vi "Main.vi"() -> ()   [LabVIEW 2014]
doc: "The boiler controller allows a user to start and shut down a boiler.\n\nUse the Reset, Start, and Light Pilot controls to sequentially start the boiler. \nUse the Fuel Control Valve to change the flow of fuel into the boiler. \nUse the Stop Boiler button to shut down the boiler. \nTo shut down the system or in the event of an emergency, use the Emergency Stop button to close the application completely."
uses:
  controls/MHL Data.ctl
  controls/MHL UI Data.ctl
  controls/MHL Status.ctl
  controls/MHL References.ctl
  controls/MHL Configuration.ctl
  support/Boiler System Globals.vi
  <vilib>/Utility/error.llb/Error Cluster From Error Code.vi
  <vilib>/ErrorRing/Error Ring.xnode
  support/Message Queue/Message Queue.lvlib
  support/User Event - Stop/User Event - Stop.lvlib
  Controller/Controller.lvlib
  Boiler/Boiler.lvlib
panel:
  in  "Fuel Control Valve":u32(slide) min=10 max=75 scale=10.0..75.0
  in  "Stop Boiler":bool
  in  "Light Pilot":bool
  out "Forced Draft Fan":bool
  out "Pilot":bool
  out "Pilot Gas Valve":bool
  out "Primary Fan":bool
  out "Status":string
  in  "Start":bool
  in  "Reset":bool
  in  "Emergency Stop":bool
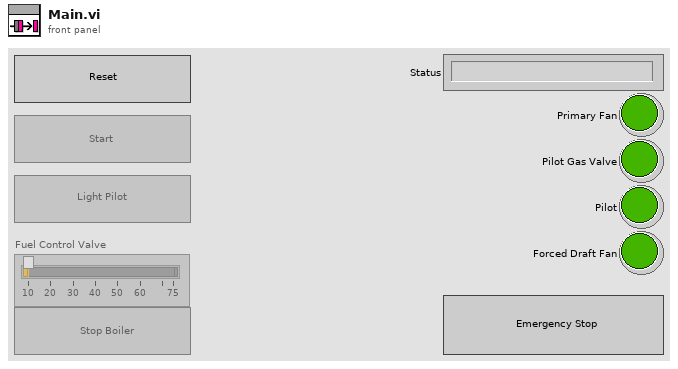
[diagram p1: front panel]
types:
  T1 = typedef "MHL Data.ctl" = cluster{"MHL User Interface Data":T2, "MHL References":T4, "MHL Configuration":T5}
  T2 = typedef "MHL UI Data.ctl" = cluster{"Status":string, "Fuel Control Valve":u32, "Primary Fan":bool, "Pilot Gas Valve":bool, "Pilot":bool, "Forced Draft Fan":bool, "MHL Status":T3}
  T3 = typedef "MHL Status.ctl" = enum16{"Lockout", "Ready", "Pre-Purge", "Pre-Purge Complete", "Pilot On", "Boiler Running", "Shutdown", "Purge"}
  T4 = typedef "MHL References.ctl" = cluster{"Reset Ref":refnum<vi>, "Start Ref":refnum<vi>, "Light Pilot Ref":refnum<vi>, "Stop Boiler Ref":refnum<vi>, "Fuel Control Valve Ref":refnum<vi>}
  T5 = typedef "MHL Configuration.ctl" = cluster{"Fuel Control Valve Maximum":dbl, "Fuel Control Valve Minimum":dbl}
  T6 = typedef "Configuration Data.ctl" = cluster{"MHL Configuration":T5, "Controller Configuration":T7, "Boiler Configuration":T8}
  T7 = typedef "Controller.lvlib/Controller Configuration.ctl" = cluster{"Purge Time":u32, "Flame Threshold":u32}
  T8 = typedef "Boiler.lvlib/Boiler Configuration.ctl" = cluster{"Pilot Increment (ms)":u32, "Pilot Decrement (ms)":u32}
  T9 = typedef "Notifiers.ctl" = cluster{"Handshake":refnum<notifier>, "Flame Level":refnum<notifier>, "Controller Exit":refnum<notifier>, "Boiler Exit":refnum<notifier>}
  T10 = typedef "Message Queue.lvlib/All Message Queues.ctl" = cluster{"MHL":refnum<queue>, "Boiler Controller":refnum<queue>, "Boiler":refnum<queue>}
  T11 = enum16{"open", "replace", "create", "open or create", "replace or create", "replace or create with confirmation"}
  T12 = enum32{"invalid app kind", "Development System", "Run Time System", "Student Edition", "Embedded LabVIEW", "Evaluation", "Custom"}
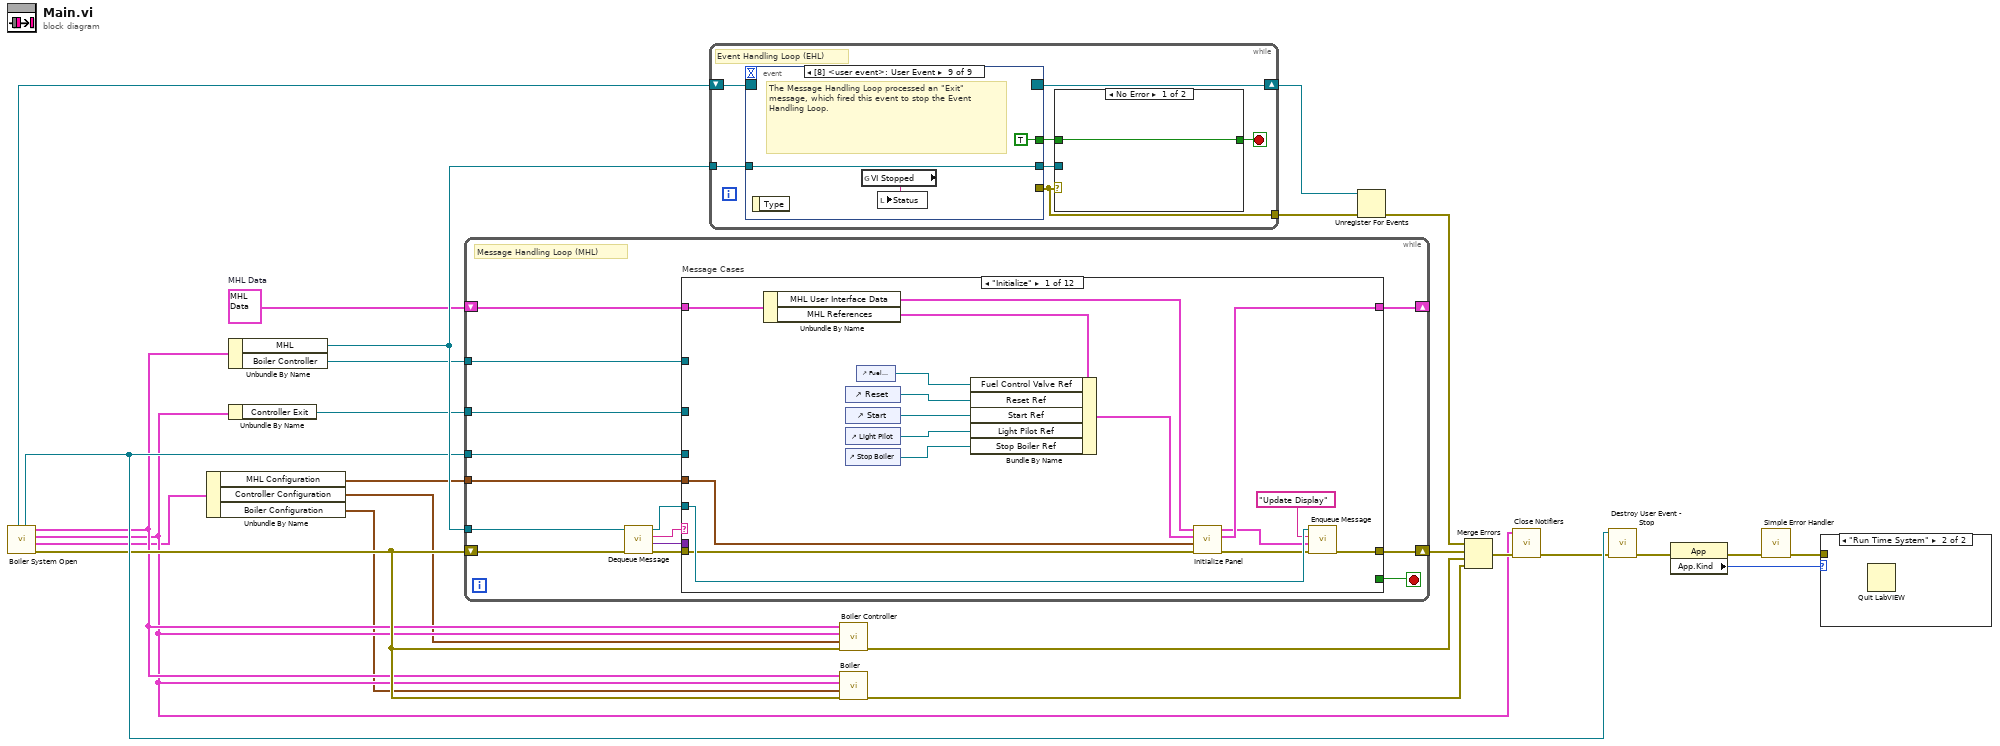
[diagram p0: block diagram]
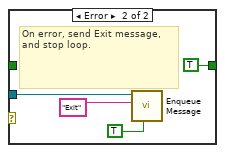
[diagram p3: hidden frame]
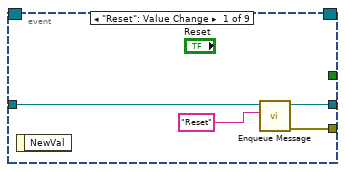
[diagram p4: hidden frame]
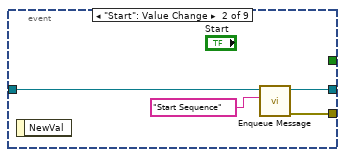
[diagram p5: hidden frame]
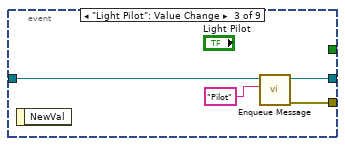
[diagram p6: hidden frame]
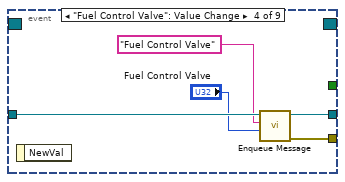
[diagram p7: hidden frame]
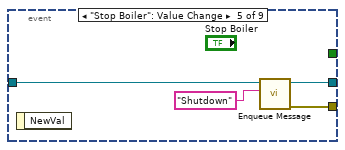
[diagram p8: hidden frame]
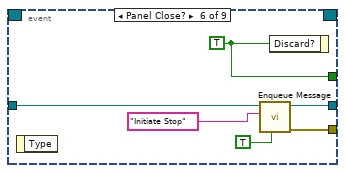
[diagram p9: hidden frame]
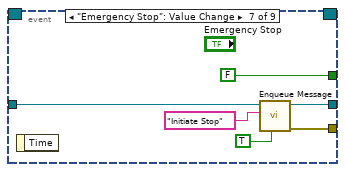
[diagram p10: hidden frame]
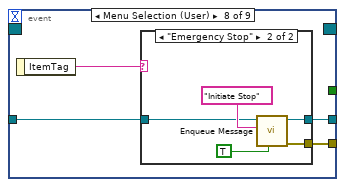
[diagram p11: hidden frame]
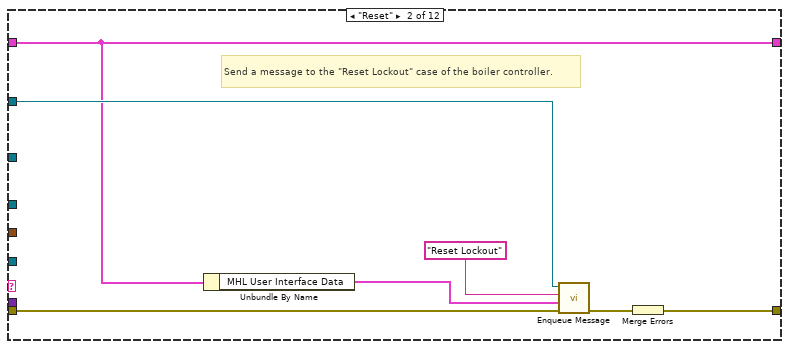
[diagram p13: hidden frame]
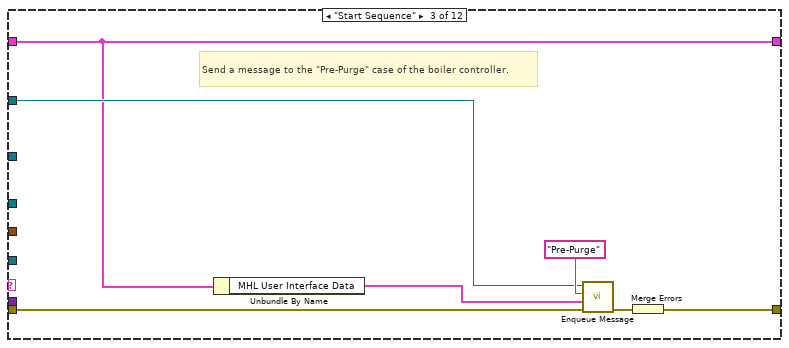
[diagram p14: hidden frame]
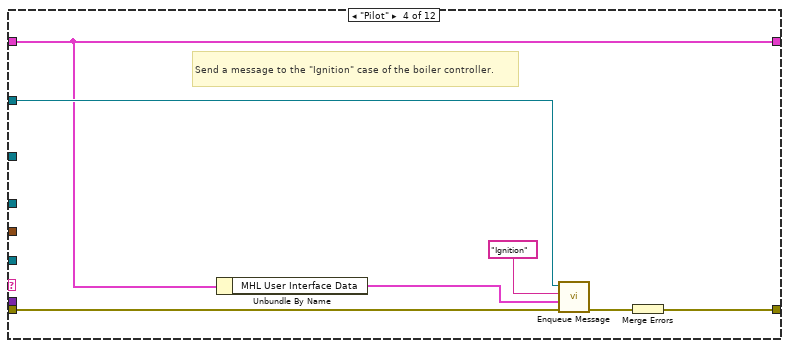
[diagram p15: hidden frame]
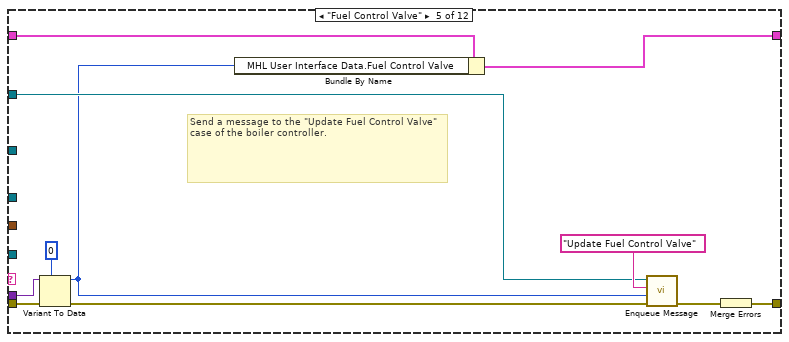
[diagram p16: hidden frame]
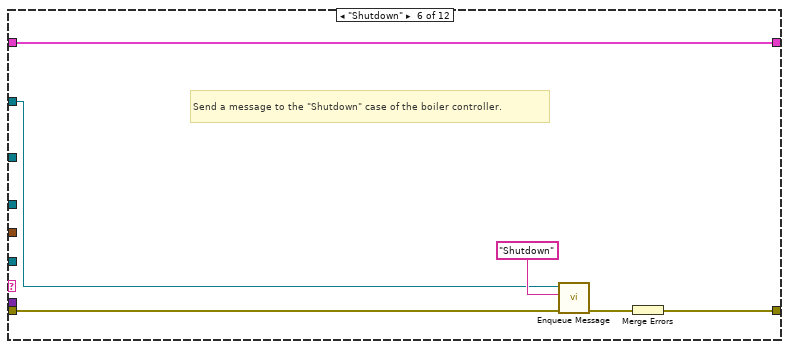
[diagram p17: hidden frame]
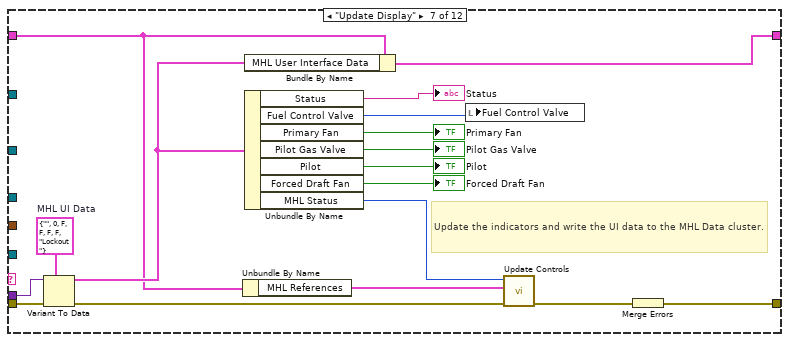
[diagram p18: hidden frame]
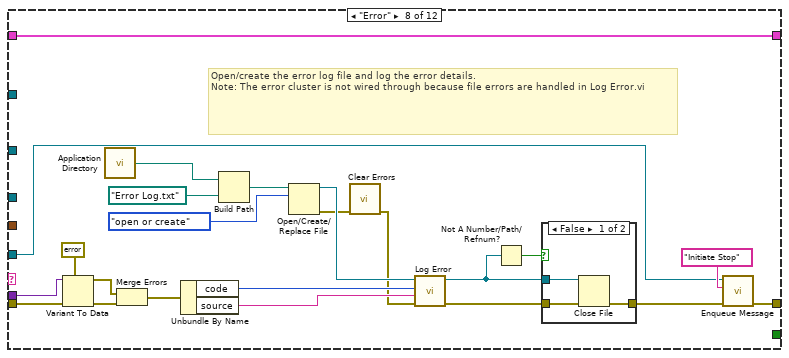
[diagram p19: hidden frame]
diagram:
  w19 = T1 {"MHL User Interface Data"={"Status"="", "Fuel Control Valve"=0, "Primary Fan"=FALSE, "Pilot Gas Valve"=FALSE, "Pilot"=FALSE, "Forced Draft Fan"=FALSE, "MHL Status"=enum."Lockout"}, "MHL References"={"Reset Ref"=refnum, "Start Ref"=refnum, "Light Pilot Ref"=refnum, "Stop Boiler Ref"=refnum, "Fuel Control Valve Ref"=refnum}, "MHL Configuration"={"Fuel Control Valve Maximum"=0.0, "Fuel Control Valve Minimum"=0.0}}  # MHL Data
  n1 = call "Boiler System Open.vi"() -> ("error out"=w10:errorcluster, "Configuration Data"=w4:T6, "Notifiers"=w5:T9, "Message Queues"=w9:T10, "User Event - Stop"=w12:refnum<user-event>, "Stop Event Registration Refnum"=w13:refnum<event-registration>)  [unwired: 6 in]
  n2 = Unbundle By Name(w4) -> ("MHL Configuration"=w3:T5, "Controller Configuration"=w2:T7, "Boiler Configuration"=w1:T8)
  n3 = Unbundle By Name(w9) -> ("MHL"=w24:refnum<queue>, "Boiler Controller"=w17:refnum<queue>)
  n4 = Unbundle By Name(w5) -> ("Controller Exit"=w11:refnum<notifier>)
  n5 = while {
    tunnel: w24 -> [w29]
    shift-right: [w38] -> _
    shift-left: w19 -> [w39]
    tunnel: w12 -> [w35]
    shift-right: [w36] -> w25
    shift-left: w10 -> [w34]
    tunnel: w17 -> [w28]
    tunnel: w11 -> [w27]
    tunnel: w3 -> [w26]
    stop <- w37 stop-if-true
    # "Message Handling Loop (MHL)"
    n6 = call "Dequeue Message.vi"("error in (no error)"=w34, "Message Queue"=w29) -> ("error out"=w33:errorcluster, "Message Data"=w31:variant, "Message"=w32:string, "dup Message Queue"=w30:refnum<queue>)  [unwired: 6 in]
    n7 = case "Message Cases" shown="\"Initialize\"" w32 {
      selector: w32 -> [_ _ _ _ _ _ _ _ _ _ _ w172]
      tunnel: w30 -> [w49 _ _ _ _ _ _ w120 w141 w148 w170 _]
      tunnel: w33 -> [w43 w62 w69 w76 w84 w92 w110 w118 w146 w150 w163 _]
      tunnel: [w50 w63 w70 w77 w88 w93 w111 w116 w143 w149 w166 w171] -> w36
      tunnel: w39 -> [w51 w58 w65 w72 w79 w94 w96 w134 w145 w154 w169 w173]
      tunnel: [w41 w58 w65 w72 w78 w94 w100 w134 w145 w154 w169 w173] -> w38
      tunnel: [_ _ _ _ _ _ _ _ _ _ TRUE _] -> w37
      tunnel: w31 -> [_ _ _ _ w82 _ w109 w117 _ _ _ _]
      tunnel: w35 -> [_ _ _ _ _ _ _ _ _ _ w165 _]
      tunnel: w28 -> [_ w59 w66 w73 w85 w89 _ _ w142 _ _ _]
      tunnel: w27 -> [_ _ _ _ _ _ _ _ _ w147 _ _]
      tunnel: w26 -> [w47 _ _ _ _ _ _ _ _ _ _ _]
      frame "Initialize" {
        n8 = Unbundle By Name(w51) -> ("MHL User Interface Data"=w44:T2, "MHL References"=w45:T4)
        n9 = control-ref of="Reset"() -> (w53:refnum<vi>)
        n10 = control-ref of="Start"() -> (w54:refnum<vi>)
        n11 = control-ref of="Light Pilot"() -> (w55:refnum<vi>)
        n12 = control-ref of="Stop Boiler"() -> (w56:refnum<vi>)
        n13 = control-ref of="Fuel Control Valve"() -> (w52:refnum<vi>)
        n14 = Bundle By Name(cluster=w45, "Fuel Control Valve Ref"=w52, "Reset Ref"=w53, "Start Ref"=w54, "Light Pilot Ref"=w55, "Stop Boiler Ref"=w56) -> (w46:T4)
        n15 = call "Initialize Panel.vi"("error in"=w43, "MHL Configuration"=w47, "MHL References"=w46, "MHL UI Data in"=w44) -> ("error out"=w42:errorcluster, "MHL Data out"=w41:T1, "MHL UI Data out"=w40:T2)  [unwired: 5 in]
        n16 = call "Enqueue Message.vi"("error in (no error)"=w42, "Message Data"=w40, "Message"="Update Display", "Message Queue"=w49) -> ("error out"=w50:errorcluster)  [unwired: 6 in, 1 out]
      }
      frame "Reset" {
        # "Send a message to the \"Reset Lockout\" case of the boiler controller."
        n17 = Unbundle By Name(w58) -> ("MHL User Interface Data"=w57:T2)
        n18 = call "Enqueue Message.vi"("error in (no error)"=w62, "Message Data"=w57, "Message"="Reset Lockout", "Message Queue"=w59) -> ("error out"=w61:errorcluster)  [unwired: 6 in, 1 out]
        n19 = Merge Errors(w61) -> (w63:errorcluster)
      }
      frame "Start Sequence" {
        # "Send a message to the \"Pre-Purge\" case of the boiler controller."
        n20 = Unbundle By Name(w65) -> ("MHL User Interface Data"=w64:T2)
        n21 = call "Enqueue Message.vi"("error in (no error)"=w69, "Message Data"=w64, "Message"="Pre-Purge", "Message Queue"=w66) -> ("error out"=w68:errorcluster)  [unwired: 6 in, 1 out]
        n22 = Merge Errors(w68) -> (w70:errorcluster)
      }
      frame "Pilot" {
        # "Send a message to the \"Ignition\" case of the boiler controller."
        n23 = Unbundle By Name(w72) -> ("MHL User Interface Data"=w71:T2)
        n24 = call "Enqueue Message.vi"("error in (no error)"=w76, "Message Data"=w71, "Message"="Ignition", "Message Queue"=w73) -> ("error out"=w75:errorcluster)  [unwired: 6 in, 1 out]
        n25 = Merge Errors(w75) -> (w77:errorcluster)
      }
      frame "Fuel Control Valve" {
        # "Send a message to the \"Update Fuel Control Valve\" case of the boiler controller."
        n26 = Variant To Data(error in=w84, type=u32 0 ("Fuel Control Valve"), Variant=w82) -> (data=w80:u32, error out=w83:errorcluster)
        n27 = Bundle By Name(cluster=w79, "MHL User Interface Data.Fuel Control Valve"=w80) -> (w78:T1)
        n28 = call "Enqueue Message.vi"("error in (no error)"=w83, "Message Data"=w80, "Message"="Update Fuel Control Valve", "Message Queue"=w85) -> ("error out"=w87:errorcluster)  [unwired: 6 in, 1 out]
        n29 = Merge Errors(w87) -> (w88:errorcluster)
      }
      frame "Shutdown" {
        # "Send a message to the \"Shutdown\" case of the boiler controller."
        n30 = call "Enqueue Message.vi"("error in (no error)"=w92, "Message"="Shutdown", "Message Queue"=w89) -> ("error out"=w91:errorcluster)  [unwired: 7 in, 1 out]
        n31 = Merge Errors(w91) -> (w93:errorcluster)
      }
      frame "Update Display" {
        w108 = T2 {"Status"="", "Fuel Control Valve"=0, "Primary Fan"=FALSE, "Pilot Gas Valve"=FALSE, "Pilot"=FALSE, "Forced Draft Fan"=FALSE, "MHL Status"=enum."Lockout"}  # MHL UI Data
        # "Update the indicators and write the UI data to the MHL Data cluster."
        n32 = Variant To Data(error in=w110, type=w108, Variant=w109) -> (data=w101:T2, error out=w99:errorcluster)
        n33 = Unbundle By Name(w96) -> ("MHL References"=w95:T4)
        n34 = Bundle By Name(cluster=w96, "MHL User Interface Data"=w101) -> (w100:T1)
        n35 = Unbundle By Name(w101) -> ("Status"=→"Status":string, "Fuel Control Valve"=w106:u32, "Primary Fan"=→"Primary Fan":bool, "Pilot Gas Valve"=→"Pilot Gas Valve":bool, "Pilot"=→"Pilot":bool, "Forced Draft Fan"=→"Forced Draft Fan":bool, "MHL Status"=w97:T3)
        n36 = local write "Fuel Control Valve"(w106) -> ()
        n37 = call "Update Controls.vi"("error in"=w99, "MHL References"=w95, "MHL Status"=w97) -> ("error out"=w98:errorcluster)  [unwired: 8 in]
        n38 = Merge Errors(w98) -> (w111:errorcluster)
      }
      frame "Error" {
        # "Open/create the error log file and log the error details.\nNote: The error cluster is not wired through because file errors are handled in Log Error.vi"
        n39 = Variant To Data(error in=w118, type=errorcluster {"status"=FALSE, "code"=0, "source"=""} ("error out"), Variant=w117) -> (data=w130:errorcluster, error out=w131:errorcluster)
        n40 = call <vilib>:"Application Directory.vi"() -> ("Application Directory"=w128:path)
        n41 = Merge Errors(w130, w131) -> (w129:errorcluster)
        n42 = Unbundle By Name(w129) -> ("code"=w123:i32, "source"=w122:string)
        n43 = Build Path(base path=w128, name or relative path=path "Error Log.txt") -> (appended path=w127:path)
        n44 = Open/Create/Replace File(file path (use dialog)=w127, operation (0:open)=T11."open or create") -> (refnum out=w125:refnum<file>, error out=w113:errorcluster)  [unwired: 4 in, 1 out]
        n45 = call <vilib>:"Clear Errors.vi"("error in (no error)"=w113) -> ("error out"=w112:errorcluster)  [unwired: 5 in, 1 out]
        n46 = call "Log Error.vi"("error in"=w112, "Source"=w122, "Code"=w123, "Error Log Refnum In"=w125) -> ("error out"=w124:errorcluster, "Error Log Refnum Out"=w115:refnum<file>)  [unwired: 6 in]
        n47 = Not A Number/Path/Refnum?(number/path/refnum=w115) -> (NaN/Path/Refnum?=w114:bool)
        n48 = case shown="False" w114 {
          tunnel: w124 -> [w137 w138]
          tunnel: w115 -> [w136 _]
          tunnel: [w135 w138] -> w121
          frame False {
            n49 = Close File(refnum=w136, error in=w137) -> (error out=w135:errorcluster)  [unwired: 1 out]
          }
          frame True {
          }
        }
        n50 = call "Enqueue Message.vi"("error in (no error)"=w121, "Message"="Initiate Stop", "Message Queue"=w120) -> ("error out"=w116:errorcluster)  [unwired: 7 in, 1 out]
      }
      frame "Initiate Stop" {
        # "When stopping, first send a message to stop the boiler controller. Then wait for the boiler and boiler controller to exit."
        n51 = call "Enqueue Message.vi"("error in (no error)"=w146, "Message"="Exit", "Message Queue"=w142) -> ("error out"=w144:errorcluster)  [unwired: 7 in, 1 out]
        n52 = call "Enqueue Message.vi"("error in (no error)"=w144, "Message"="Wait on Boiler Exit", "Message Queue"=w141) -> ("error out"=w143:errorcluster)  [unwired: 7 in, 1 out]
      }
      frame "Wait on Boiler Exit" {
        # "Monitor the boiler controller to determine if it has completed its Exit. Wait 10 milliseconds for the boiler controller to respond. \nIf the notification does not occur, then enqueue another Wait on Boiler Exit message.\nIf the notification occurs, then exit the Message Handling Loop."
        n53 = Wait on Notification(notifier=w147, timeout in ms (-1)=10, error in (no error)=w150) -> (timed out?=w152:bool, error out=w151:errorcluster)  [unwired: 1 in, 2 out]
        n54 = case shown="True" w152 {
          tunnel: w151 -> [w158 w162]
          tunnel: w148 -> [w157 w160]
          tunnel: [w155 w161] -> w149
          frame False {
            n55 = call "Enqueue Message.vi"("error in (no error)"=w158, "Message"="Exit", "Message Queue"=w157) -> ("error out"=w155:errorcluster)  [unwired: 7 in, 1 out]
          }
          frame True {
            n56 = call "Enqueue Message.vi"("error in (no error)"=w162, "Message"="Wait on Boiler Exit", "Message Queue"=w160) -> ("error out"=w161:errorcluster)  [unwired: 7 in, 1 out]
          }
        }
      }
      frame "Exit" {
        # "Stop the VI"
        # "Release the message queue reference"
        n57 = call "Fire User Event - Stop.vi"("User Event - Stop"=w165) -> ("error out"=w164:errorcluster)  [unwired: 10 in]
        n58 = Release Queue(queue=w170, error in (no error)=w163) -> (error out=w167:errorcluster)  [unwired: 1 in, 2 out]
        n59 = Merge Errors(w164, w167) -> (w166:errorcluster)
      }
      frame Default {
        # "'Default' case only runs if there is a message that isn't defined in any of the other cases.  Output a programming error."
        n60 = xnode "Error Ring"("parameter 0"=w172) -> ("error out"=w171:errorcluster)
      }
    }
  }
  n61 = while {
    tunnel: w24 -> [w187]
    tunnel: [w183] -> w21
    shift-right: [w181] -> w20
    shift-left: w13 -> [w182]
    stop <- w185 stop-if-true
    # "Event Handling Loop (EHL)"
    n62 = event shown="[8] <user event>: User Event" {
      selector: w182 -> [_ _ _ _ _ _ _ _ _]
      dyn-events: [_ _ _ _ _ _ _ _ _] -> w181
      timeout: _ -> [_ _ _ _ _ _ _ _ _]
      tunnel: [_ _ _ _ _ w219 FALSE ("Discard?") _ TRUE ("Discard?")] -> w186
      tunnel: w187 -> [w196 w200 w204 w209 w213 w218 w225 w228 w238]
      tunnel: [w195 w198 w202 w207 w211 w217 w224 w226 _] -> w183
      tunnel: [w194 w199 w203 w208 w212 w216 w222 w227 w238] -> w184
      event "Reset": Value Change {
        n63 = event-data() -> ()  [unwired: 1 in, 1 out]
        n64 = call "Enqueue Message.vi"("Message"="Reset", "Message Queue"=w196) -> ("error out"=w195:errorcluster, "dup Message Queue"=w194:refnum<queue>)  [unwired: 8 in]
      }
      event "Start": Value Change {
        n65 = event-data() -> ()  [unwired: 1 in, 1 out]
        n66 = call "Enqueue Message.vi"("Message"="Start Sequence", "Message Queue"=w200) -> ("error out"=w198:errorcluster, "dup Message Queue"=w199:refnum<queue>)  [unwired: 8 in]
      }
      event "Light Pilot": Value Change {
        n67 = event-data() -> ()  [unwired: 1 in, 1 out]
        n68 = call "Enqueue Message.vi"("Message"="Pilot", "Message Queue"=w204) -> ("error out"=w202:errorcluster, "dup Message Queue"=w203:refnum<queue>)  [unwired: 8 in]
      }
      event "Fuel Control Valve": Value Change {
        n69 = event-data() -> ()  [unwired: 1 in, 1 out]
        n70 = call "Enqueue Message.vi"("Message Data"="Fuel Control Valve", "Message"="Fuel Control Valve", "Message Queue"=w209) -> ("error out"=w207:errorcluster, "dup Message Queue"=w208:refnum<queue>)  [unwired: 7 in]
      }
      event "Stop Boiler": Value Change {
        n71 = event-data() -> ()  [unwired: 1 in, 1 out]
        n72 = call "Enqueue Message.vi"("Message"="Shutdown", "Message Queue"=w213) -> ("error out"=w211:errorcluster, "dup Message Queue"=w212:refnum<queue>)  [unwired: 8 in]
      }
      event Panel Close? {
        w219 = TRUE ("Discard?")
        n73 = event-data() -> ()  [unwired: 1 in, 1 out]
        n74 = call "Enqueue Message.vi"("Priority Message? (F)"=TRUE, "Message"="Initiate Stop", "Message Queue"=w218) -> ("error out"=w217:errorcluster, "dup Message Queue"=w216:refnum<queue>)  [unwired: 7 in]
        n75 = event-data("Discard?"=w219) -> ()  [unwired: 1 in, 1 out]
      }
      event "Emergency Stop": Value Change {
        n76 = event-data() -> ()  [unwired: 1 in, 1 out]
        n77 = call "Enqueue Message.vi"("Priority Message? (F)"=TRUE, "Message"="Initiate Stop", "Message Queue"=w225) -> ("error out"=w224:errorcluster, "dup Message Queue"=w222:refnum<queue>)  [unwired: 7 in]
      }
      event Menu Selection (User) {
        n78 = event-data() -> ("ItemTag"=w229:string)  [unwired: 1 in]
        n79 = case shown="\"Emergency Stop\"" w229 {
          tunnel: w228 -> [w230 w233]
          tunnel: [w230 w232] -> w227
          tunnel: [_ w231] -> w226
          frame Default {
          }
          frame "Emergency Stop" {
            n80 = call "Enqueue Message.vi"("Priority Message? (F)"=TRUE, "Message"="Initiate Stop", "Message Queue"=w233) -> ("error out"=w231:errorcluster, "dup Message Queue"=w232:refnum<queue>)  [unwired: 7 in]
          }
        }
      }
      event User Event {
        # "The Message Handling Loop processed an \"Exit\" message, which fired this event to stop the Event Handling Loop."
        n81 = event-data() -> ()  [unwired: 1 in, 1 out]
        n82 = global read "Boiler System Globals.vi" "VI Stopped"() -> (w236:string)
        n83 = local write "Status"(w236) -> ()
      }
    }
    n84 = case shown="No Error" w183 {
      tunnel: [w188 TRUE ("Discard?")] -> w185
      tunnel: w186 -> [w188 _]
      tunnel: w184 -> [_ w191]
      frame No Error {
      }
      frame Error {
        # "On error, send Exit message, and stop loop."
        n85 = call "Enqueue Message.vi"("Priority Message? (F)"=TRUE, "Message"="Exit", "Message Queue"=w191) -> ()  [unwired: 7 in, 2 out]
      }
    }
  }
  n86 = call "Boiler Controller.vi"("error in"=w10, "Controller Configuration"=w2, "Notifiers"=w5, "Message Queues"=w9) -> ("error out"=w18:errorcluster)  [unwired: 7 in]
  n87 = call "Boiler.vi"("error in"=w10, "Boiler Configuration"=w1, "Notifiers"=w5, "Message Queues"=w9) -> ("error out"=w8:errorcluster)  [unwired: 7 in]
  n88 = Unregister For Events(event registration refnum=w20, error in=w21) -> (error out=w22:errorcluster)
  n89 = Merge Errors(w22, w25, w18, w8) -> (w7:errorcluster)
  n90 = call "Close Notifiers.vi"("error in"=w7, "Notifiers"=w5) -> ("error out"=w6:errorcluster)  [unwired: 9 in]
  n91 = call "Destroy User Event - Stop.vi"("error in (no error)"=w6, "User Event - Stop"=w12) -> ("error out"=w23:errorcluster)  [unwired: 9 in]
  n92 = property class="App"(error in=w23) -> (error out=w16:errorcluster, "App.Kind"=w15:T12)  [unwired: 1 in, 1 out]
  n93 = call <vilib>:"Simple Error Handler.vi"("error in (no error)"=w16) -> ("error out"=w14:errorcluster)  [unwired: 4 in, 4 out]
  n94 = case shown="\"Run Time System\"" w15 {
    tunnel: w14 -> [_ _]
    frame Default {
    }
    frame "Run Time System" {
      n95 = Quit LabVIEW() -> ()  [unwired: 1 in]
    }
  }
